vi "Find largest Network from Candidate.vi"(10 "Candidate Network":set{string}(c389), 11 "NetAn in":refnum<class "NetAn.lvclass">) -> (2 "Largest Network":set{string}(c389), 3 "NetAn out":refnum<class "NetAn.lvclass">)   [LabVIEW 2020, in "NetAn.lvclass"]
uses:
  NetAn.lvclass
  Global 1.vi
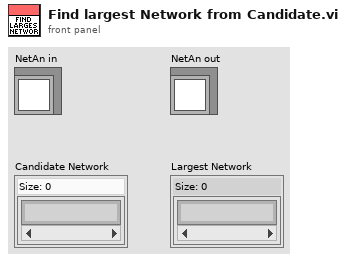
[diagram p1: front panel]
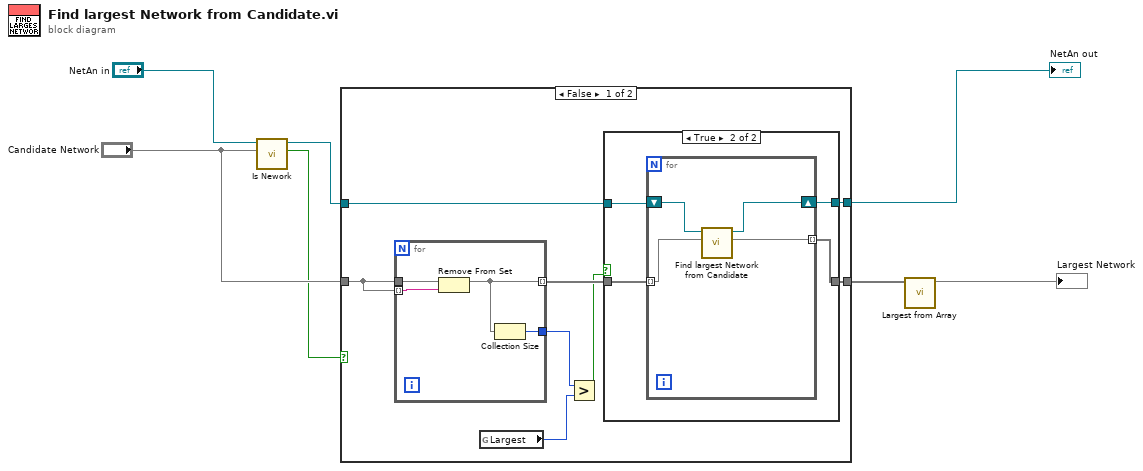
[diagram p0: block diagram]
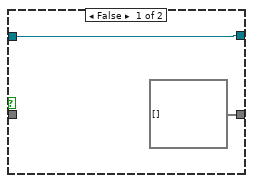
[diagram p2: hidden frame]
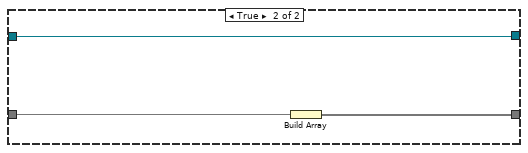
[diagram p3: hidden frame]
diagram:
  n1 = call "Is Nework.vi"("Set"="Candidate Network", "NetAn in"="NetAn in") -> ("Is network"=w1:bool, "NetAn out"=w3:refnum<class "NetAn.lvclass">)  [unwired: 8 in]
  n2 = case shown="False" w1 {
    tunnel: "Candidate Network" -> [w13 w32]
    tunnel: [w11 w30] -> w2
    tunnel: w3 -> [w15 w31]
    tunnel: [w14 w31] -> w7
    frame False {
      n3 = for {
        tunnel: w13 -> [w28] mode=indexing
        tunnel: w13 -> [w29]
        tunnel: [w27] -> w12 mode=indexing
        tunnel: [w26] -> w8
        n4 = Remove From Set(10:w28, 11:w29) -> (3:w27:set{string})  [unwired: 1 out]
        n5 = Collection Size(1:w27) -> (0:w26:i32)
      }
      n6 = global read "Global 1.vi" "Largest"() -> (w10:i32)
      n7 = Greater?(x=w8, y=w10) -> (0:w9:bool)
      n8 = case shown="True" w9 {
        tunnel: w15 -> [w17 w21]
        tunnel: [w17 w20] -> w14
        tunnel: w12 -> [_ w19]
        tunnel: [set{string}[] [] w18] -> w11
        frame False {
        }
        frame True {
          n9 = for {
            shift-right: [w24] -> w20
            shift-left: w21 -> [w25]
            tunnel: w19 -> [w23] mode=indexing
            tunnel: [w22] -> w18 mode=indexing
            n10 = call "Find largest Network from Candidate.vi"("Candidate Network"=w23, "NetAn in"=w25) -> ("Largest Network"=w22:set{string}, "NetAn out"=w24:refnum<class "NetAn.lvclass">)  [unwired: 8 in]
          }
        }
      }
    }
    frame True {
      n11 = Build Array(w32) -> (w30:set{string}[])
    }
  }
  "NetAn out" <- w7
  n12 = call "Largest from Array.vi"("Array"=w2) -> ("Largest Network"=→"Largest Network":set{string})  [unwired: 10 in]
